vi "View  beam possitions.vi"(8 "error in (no error)":errorcluster, 10 "Beam on cup":T1(radio), 11 "Lifter_motor in":refnum<class "Lifter_motor.lvclass">) -> (0 "error out":errorcluster, 2 "Location (mm)":dbl, 3 "Lifter_motor out":refnum<class "Lifter_motor.lvclass">)   [LabVIEW 2019, in "Lifter_motor.lvclass"]
uses:
  Lifter_motor.lvclass
  Lifter_motor.lvclass/Lifter_motor.ctl
panel:
  out "locations":dbl[](array[numeric])
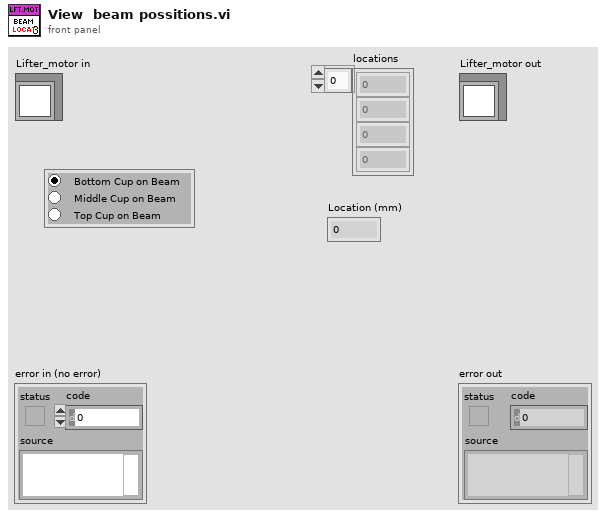
[diagram p1: front panel]
types:
  T1 = enum32{"Bottom Cup on Beam", "Middle Cup on Beam", "Top Cup on Beam"}
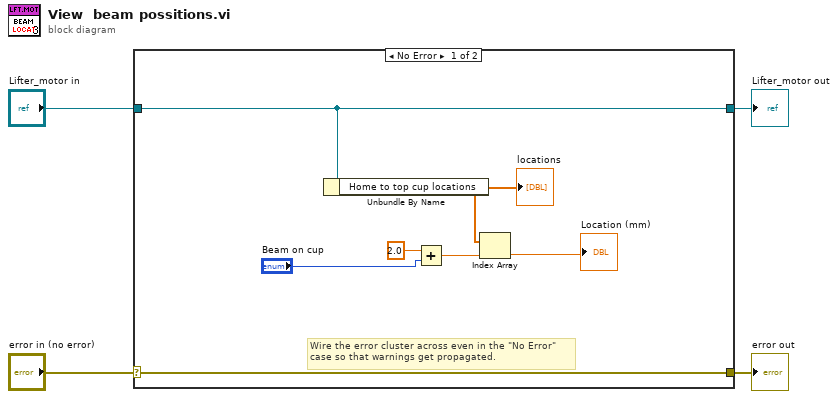
[diagram p0: block diagram]
diagram:
  n1 = case shown="No Error" "error in (no error)" {
    selector: "error in (no error)" -> [w11 w13]
    tunnel: [w11 w13] -> w3
    tunnel: [w10 w12] -> w1
    tunnel: "Lifter_motor in" -> [w10 w12]
    frame No Error {
      # "Wire the error cluster across even in the \"No Error\"\ncase so that warnings get propagated."
      n2 = Unbundle By Name(w10) -> ("Home to top cup locations"=w9:dbl[])
      "locations" <- w9
      n3 = Add(x=2.0, y="Beam on cup") -> (x+y=w6:dbl)
      n4 = Index Array(array=w9, index=w6) -> (element=→"Location (mm)":dbl)
    }
    frame Error {
    }
  }
  "error out" <- w3
  "Lifter_motor out" <- w1
